vi "EncapsulatedAutonomous.vi"   [LabVIEW 2017]
uses:
  <vilib>/Rock Robotics/Network Tables/NT Read Numeric Array.vi
  <vilib>/Rock Robotics/Network Tables/NT Read Number.vi
  <vilib>/Rock Robotics/Network Tables/NT Read Boolean.vi
  <vilib>/Rock Robotics/Network Tables/NT Write String.vi
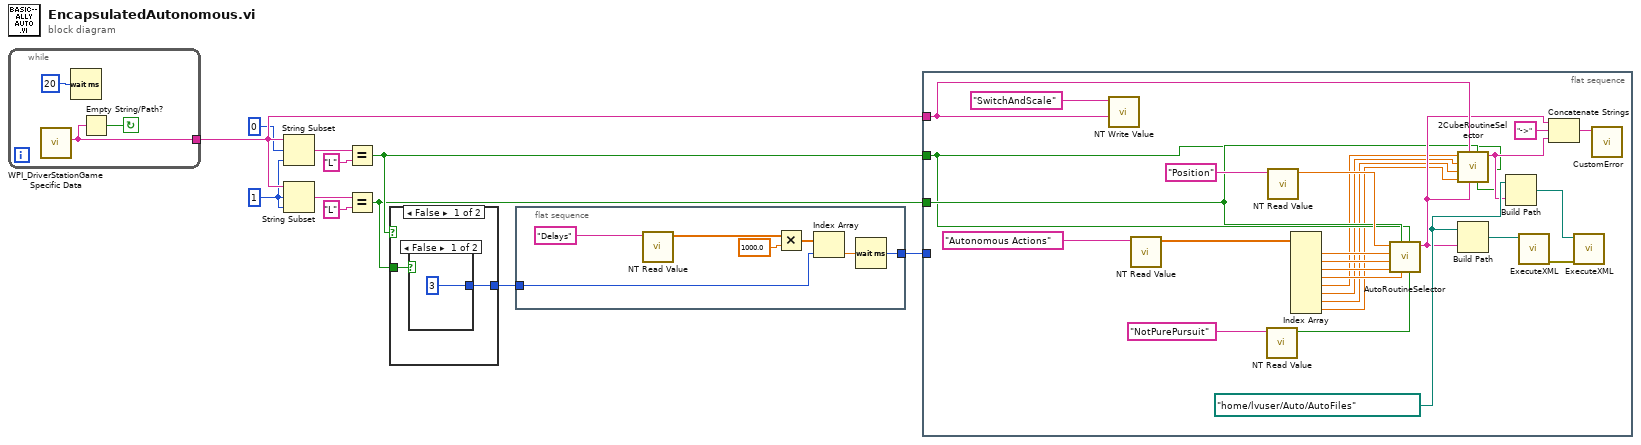
[diagram p0: block diagram]
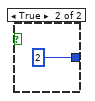
[diagram p2: hidden frame]
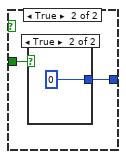
[diagram p3: hidden frame]
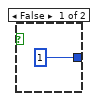
[diagram p4: hidden frame]
diagram:
  w6 = 1 ("length (rest)")
  n1 = while {
    tunnel: [w14] -> w11
    stop <- w13 continue-if-true
    n2 = call <vilib>:"WPI_DriverStationGame Specific Data.vi"() -> ("Game Specific Data"=w14:string)  [unwired: 11 in]
    n3 = Wait (ms)(milliseconds to wait=u32 20) -> ()  [unwired: 1 out]
    n4 = Empty String/Path?(string/path=w14) -> (empty?=w13:bool)
  }
  n5 = String Subset(string=w11, offset (0)=0 ("length (rest)"), length (rest)=w6) -> (substring=w9:string)
  n6 = String Subset(string=w11, offset (0)=w6, length (rest)=w6) -> (substring=w10:string)
  n7 = Equal?(x=w9, y="L") -> (x = y?=w4:bool)
  n8 = Equal?(x=w10, y="L") -> (x = y?=w3:bool)
  n9 = case shown="False" w4 {
    tunnel: w3 -> [w16 w20]
    tunnel: [w15 w19] -> w1
    frame False {
      n10 = case shown="False" w16 {
        tunnel: [3 2] -> w15
        frame False {
        }
        frame True {
        }
      }
    }
    frame True {
      n11 = case shown="True" w20 {
        tunnel: [1 0] -> w19
        frame False {
        }
        frame True {
        }
      }
    }
  }
  n12 = flat-sequence {
    tunnel: w1 -> [w24]
    tunnel: [w23] -> w2
    frame #0 {
      n13 = call-poly <vilib>:"NT Read Value.vi"("Name"="Delays") -> ("Numeric Array"=w29:dbl[])  [unwired: 9 in, 1 out]
      n14 = Multiply(x=w29, y=1000.0) -> (x*y=w26:dbl[])
      n15 = Index Array(array=w26, index=w24) -> (element=w25:dbl)
      n16 = Wait (ms)(milliseconds to wait=w25) -> (millisecond timer value=w23:u32)
    }
  }
  n17 = flat-sequence {
    tunnel: w11 -> [w52]
    tunnel: w3 -> [w38]
    tunnel: w4 -> [w37]
    tunnel: w2 -> [_]
    frame #0 {
      w51 = path "/home/lvuser/Auto/AutoFiles" ("base path")
      n18 = call-poly <vilib>:"NT Write Value.vi"("String"=w52, "Name"="SwitchAndScale") -> ()  [unwired: 9 in, 1 out]
      n19 = call-poly <vilib>:"NT Read Value.vi"("Name"="Autonomous Actions") -> ("Numeric Array"=w45:dbl[])  [unwired: 9 in, 1 out]
      n20 = call-poly <vilib>:"NT Read Value.vi"("Name"="NotPurePursuit") -> ("Boolean"=w44:bool)  [unwired: 9 in, 1 out]
      n21 = call-poly <vilib>:"NT Read Value.vi"("Name"="Position") -> ("Numeric"=w50:dbl)  [unwired: 9 in, 1 out]
      n22 = Index Array(array=w45) -> (element #1=w43:dbl, element #2=w42:dbl, element #3=w41:dbl, element #4=w40:dbl, element #5=w36:dbl, element #6=w35:dbl, element #7=w34:dbl, element #8=w33:dbl)  [unwired: 8 in]
      n23 = call "AutoRoutineSelector.vi"("NotPurePursuit"=w44, "OurSwitch"=w37, "RR"=w40, "OurScale"=w38, "RL"=w41, "LR"=w42, "LL"=w43, "Position"=w50) -> ("File Name"=w39:string)  [unwired: 3 in]
      n24 = call "2CubeRoutineSelector.vi"("Switch"=w37, "Scale"=w38, "Prior Routine File Name"=w39, "GameData"=w52, "RR"=w33, "RL"=w34, "LR"=w35, "LL"=w36) -> ("File Path"=w48:string)  [unwired: 3 in]
      n25 = Build Path(base path=w51, name or relative path=w39) -> (appended path=w32:path)
      n26 = Build Path(base path=w51, name or relative path=w48) -> (appended path=w31:path)
      n27 = call "ExecuteXML.vi"("Auto File Path"=w32) -> ("error out"=w30:errorcluster)  [unwired: 10 in]
      n28 = Concatenate Strings(w39, "->" ("string"), w48) -> (w47:string)
      n29 = call "ExecuteXML.vi"("error in (no error)"=w30, "Auto File Path"=w31) -> ()  [unwired: 9 in, 1 out]
      n30 = call "CustomError.vi"("String"=w47) -> ()  [unwired: 10 in, 1 out]
    }
  }
